vi "CheckAlarms.vi"(8 "entrée d'erreur (pas d'erreur)":errorcluster, 10 "ControlQueue":refnum<queue>, 11 "DAQmxTaskContainer en entrée":refnum<class "DAQmxTaskContainer.lvclass">) -> (0 "sortie d'erreur":errorcluster, 3 "DAQmxTaskContainer en sortie":refnum<class "DAQmxTaskContainer.lvclass">)   [LabVIEW 2015, in "DAQmxTaskContainer.lvclass"]
uses:
  DAQmxTaskContainer.lvclass
  DAQmxTaskAICurrent.lvclass/DAQmxTaskAICurrent.ctl
  DAQmxTask.lvclass
  DAQmxTaskAICurrent.lvclass
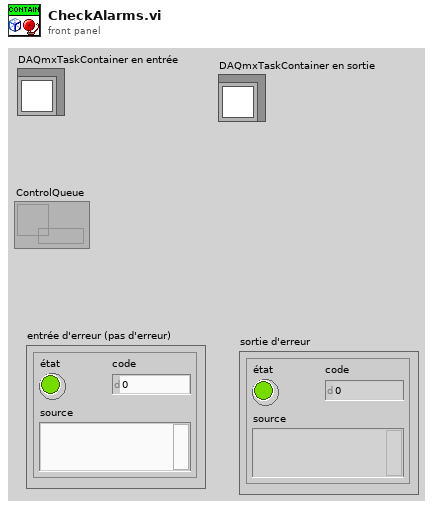
[diagram p1: front panel]
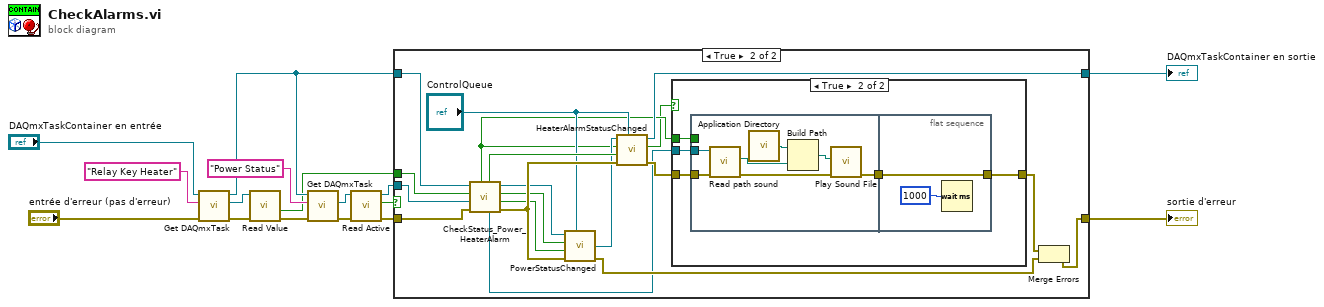
[diagram p0: block diagram]
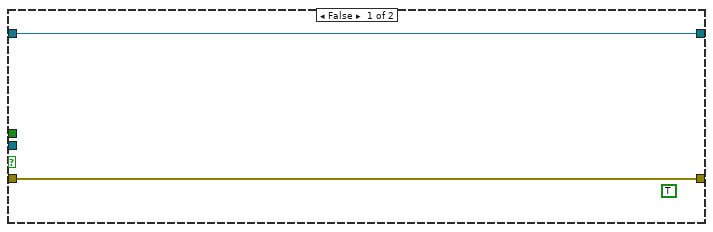
[diagram p2: hidden frame]
diagram:
  n1 = call "Get DAQmxTask.vi"("error in (no error)"="entrée d'erreur (pas d'erreur)", "Task name"="Relay Key Heater", "DAQmxTaskContainer in"="DAQmxTaskContainer en entrée") -> ("error out"=w8:errorcluster, "DAQmx Task"=w7:refnum<class "DAQmxTask.lvclass">, "DAQmxTaskContainer out"=w5:refnum<class "DAQmxTaskContainer.lvclass">)  [unwired: 6 in]
  n2 = call-dynamic "Read Value.vi"("error in (no error)"=w8, "DAQmxTask en entrée"=w7) -> ("error out"=w4:errorcluster, "Data"=w3:bool)  [unwired: 6 in, 2 out]
  n3 = call "Get DAQmxTask.vi"("error in (no error)"=w4, "Task name"="Power Status", "DAQmxTaskContainer in"=w5) -> ("error out"=w14:errorcluster, "DAQmx Task"=w13:refnum<class "DAQmxTask.lvclass">)  [unwired: 6 in, 1 out]
  n4 = call-dynamic "Read Active.vi"("error in (no error)"=w14, "DAQmxTask in"=w13) -> ("error out"=w11:errorcluster, "Active?"=w9:bool, "DAQmxTask out"=w12:refnum<class "DAQmxTask.lvclass">)  [unwired: 7 in]
  n5 = case shown="True" w9 {
    tunnel: [w17 w32] -> w16
    tunnel: [w18 w28] -> w15
    tunnel: w12 -> [_ w37]
    tunnel: w11 -> [w17 w34]
    tunnel: w5 -> [w18 w35]
    tunnel: w3 -> [_ w30]
    frame False {
      (unwired) TRUE ("First Time")
    }
    frame True {
      n6 = call "CheckStatus_Power_HeaterAlarm.vi"("entrée d'erreur (pas d'erreur)"=w34, "DAQmxTask out"=w37, "RelayKeyStatus"=w30, "DAQmxTaskContainer en entrée"=w35) -> ("sortie d'erreur"=w31:errorcluster, "PowerStatus"=w29:bool, "PowerStatusChanged"=w23:bool, "DAQmxTaskContainer en sortie"=w26:refnum<class "DAQmxTaskContainer.lvclass">, "DAQmxTaskAICurrent en sortie"=w20:refnum<class "DAQmxTaskAICurrent.lvclass">, "HeaterAlarmStatus"=w27:bool, "HeaterAlarmStatusChanged"=w21:bool)  [unwired: 1 in]
      n7 = call "PowerStatusChanged.vi"("ControlQueue"="ControlQueue", "entrée d'erreur (pas d'erreur)"=w31, "PowerStatus"=w29, "PowerStatusChanged"=w23, "DAQmxTaskContainer en entrée"=w26) -> ("sortie d'erreur"=w25:errorcluster, "DAQmxTaskContainer en sortie"=w24:refnum<class "DAQmxTaskContainer.lvclass">)  [unwired: 5 in]
      n8 = call "HeaterAlarmStatusChanged.vi"("ControlQueue"="ControlQueue", "entrée d'erreur (pas d'erreur)"=w31, "HeaterAlarmStatus"=w27, "HeaterAlarmStatusChanged"=w21, "DAQmxTaskContainer en entrée"=w24) -> ("sortie d'erreur"=w36:errorcluster, "Alarm"=w19:bool, "DAQmxTaskContainer en sortie"=w28:refnum<class "DAQmxTaskContainer.lvclass">)  [unwired: 4 in]
      n9 = case shown="True" w19 {
        tunnel: w36 -> [w38 w43]
        tunnel: [w38 w42] -> w33
        tunnel: w21 -> [_ w41]
        tunnel: w20 -> [_ w39]
        frame False {
        }
        frame True {
          n10 = flat-sequence {
            tunnel: w43 -> [w49]
            tunnel: w41 -> [_]
            tunnel: [w48] -> w40
            tunnel: w39 -> [w47]
            tunnel: [w52] -> w42
            tunnel: w40 -> [w52]
            frame #0 {
              n11 = call "Read path sound.vi"("error in (no error)"=w49, "DAQmxTaskAICurrent en entrée"=w47) -> ("error out"=w50:errorcluster, "path sound"=w45:path)  [unwired: 7 in, 1 out]
              n12 = call <vilib>:"Application Directory.vi"() -> ("Application Directory"=w46:path)
              n13 = Build Path(base path=w46, name or relative path=w45) -> (appended path=w44:path)
              n14 = call <vilib>:"Play Sound File.vi"("error in (no error)"=w50, "path"=w44) -> ("error out"=w48:errorcluster)  [unwired: 8 in, 1 out]
            }
            frame #1 {
              n15 = Wait (ms)(milliseconds to wait=u32 1000 ("attente (ms)")) -> ()  [unwired: 1 out]
            }
          }
        }
      }
      n16 = Merge Errors(w33, w25) -> (w32:errorcluster)
    }
  }
  "sortie d'erreur" <- w16
  "DAQmxTaskContainer en sortie" <- w15
